vi "Unconstrained Gaussian Peak Fit.vi"(0 "Y":dbl[](array[numeric]), 1 "initial guess":T1={"initial amplitude"=nan, "initial center"=nan, "initial standard deviation"=nan}, 5 "X":dbl[](array[numeric]), 7 "Weight":dbl[](array[numeric]), 9 "tolerance":dbl=0.0001 format="%#_3g", 11 "method":T2 items=["Least Square", "Least Absolute Residual", "Bisquare"]) -> (4 "Best Gaussian Fit":dbl[](array[numeric]), 6 "amplitude":dbl, 8 "center":dbl, 10 "standard deviation":dbl, 14 "residue":dbl, 15 "error":i32)   [LabVIEW 2017, in "NI_AALPro.lvlib"]
doc: "LabVIEW does not support the Unconstrained Gaussian Peak Fit VI. Use the Gaussian Peak Fit VI instead."
uses:
  NI_AALPro.lvlib
  Curve Fitting Criteria.ctl
panel:
  # "Gaussian Peak Fit"
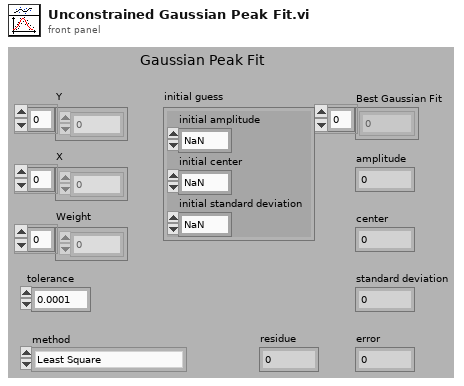
[diagram p1: front panel]
types:
  T1 = cluster{"initial amplitude":dbl, "initial center":dbl, "initial standard deviation":dbl}
  T2 = typedef "NI_AALPro.lvlib/Curve Fitting Criteria.ctl" = u16
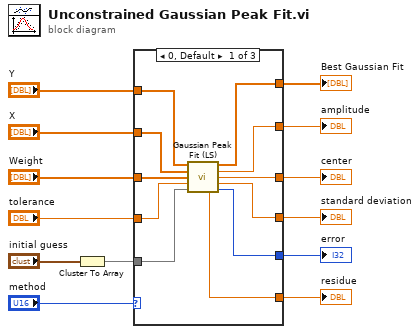
[diagram p0: block diagram]
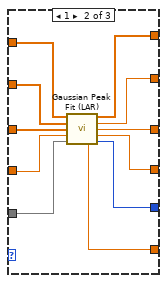
[diagram p2: hidden frame]
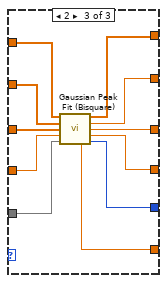
[diagram p3: hidden frame]
diagram:
  n1 = Cluster To Array(cluster="initial guess") -> (array=w2:dbl[])
  n2 = case shown="0, Default" "method" {
    tunnel: "Y" -> [w24 w35 w46]
    tunnel: "X" -> [w23 w34 w45]
    tunnel: "Weight" -> [w22 w33 w44]
    tunnel: "tolerance" -> [w21 w32 w43]
    tunnel: w2 -> [w20 w31 w42]
    tunnel: [w19 w30 w41] -> w8
    tunnel: [w18 w29 w40] -> w7
    tunnel: [w17 w28 w39] -> w6
    tunnel: [w16 w27 w38] -> w5
    tunnel: [w15 w26 w37] -> w4
    tunnel: [w14 w25 w36] -> w3
    frame 0, Default {
      n3 = call "Gaussian Peak Fit (LS).vi"("Y"=w24, "X"=w23, "Weight"=w22, "tolerance"=w21, "Initial Coefficients"=w20) -> ("Best Gaussian Fit"=w19:dbl[], "amplitude"=w18:dbl, "center"=w17:dbl, "width"=w16:dbl, "residue"=w14:dbl, "error"=w15:i32)  [unwired: 5 out]
    }
    frame 1 {
      n4 = call "Gaussian Peak Fit (LAR).vi"("Y"=w35, "X"=w34, "Weight"=w33, "tolerance"=w32, "Initial Coefficients"=w31) -> ("Best Gaussian Fit"=w30:dbl[], "amplitude"=w29:dbl, "center"=w28:dbl, "width"=w27:dbl, "residue"=w25:dbl, "error"=w26:i32)  [unwired: 5 out]
    }
    frame 2 {
      n5 = call "Gaussian Peak Fit (Bisquare).vi"("Y"=w46, "X"=w45, "Weight"=w44, "tolerance"=w43, "Initial Coefficients"=w42) -> ("Best Gaussian Fit"=w41:dbl[], "amplitude"=w40:dbl, "center"=w39:dbl, "width"=w38:dbl, "residue"=w36:dbl, "error"=w37:i32)  [unwired: 5 out]
    }
  }
  "amplitude" <- w7
  "center" <- w6
  "standard deviation" <- w5
  "error" <- w4
  "Best Gaussian Fit" <- w8
  "residue" <- w3
